vi "evalPerf.vi"(8 "error in (no error)":errorcluster, 11 "removeTempDir":bool=TRUE) -> (0 "error out":errorcluster, 3 "totalTimeInSec":dbl)   [LabVIEW 2018]
doc: "Evaluate the performance. The total used time will show on the panel."
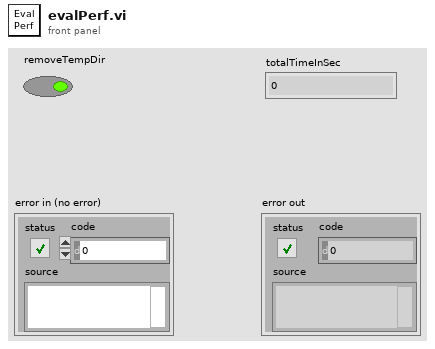
[diagram p1: front panel]
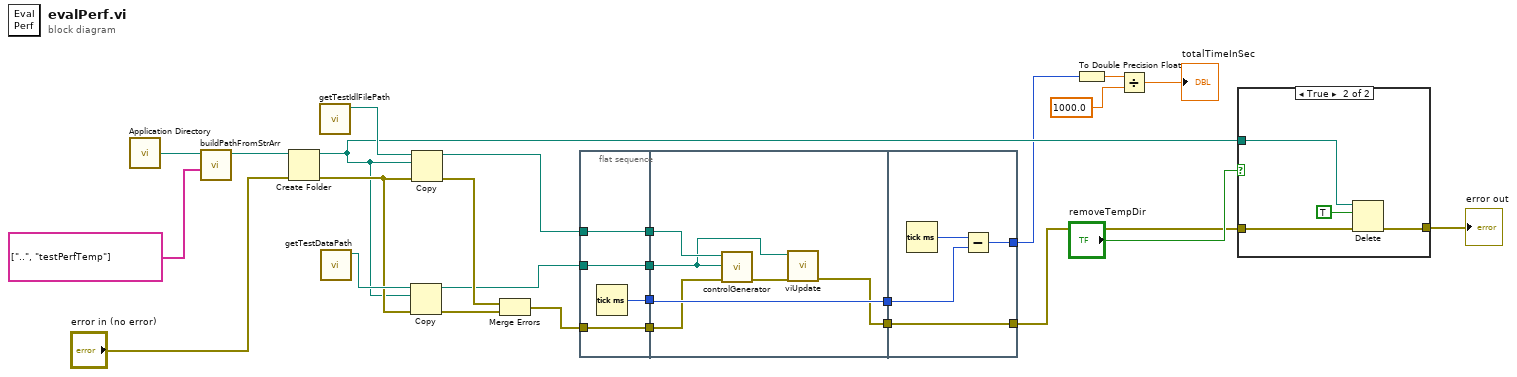
[diagram p0: block diagram]
diagram:
  n1 = call <vilib>:"Application Directory.vi"() -> ("Application Directory"=w26:path)
  n2 = call "buildPathFromStrArr.vi"("String Array"=string[] ["..", "testPerfTemp"], "Root Path"=w26) -> ("Absolute Path"=w24:path)  [unwired: 9 in]
  n3 = Create Folder(path (use dialog)=w24, error in="error in (no error)") -> (created path=w15:path, error out=w20:errorcluster)  [unwired: 1 in, 1 out]
  n4 = call "getTestIdlFilePath.vi"() -> ("testIdlPath"=w22:path)  [unwired: 11 in]
  n5 = call "getTestDataPath.vi"() -> ("testDataPath"=w21:path)  [unwired: 11 in]
  n6 = Copy(8:w20, 10:w15, 11:w21) -> (0:w18:errorcluster, 3:w8:path)  [unwired: 2 in, 1 out]
  n7 = Copy(8:w20, 10:w15, 11:w22) -> (0:w19:errorcluster, 3:w10:path)  [unwired: 2 in, 1 out]
  n8 = Merge Errors(w19, w18) -> (w11:errorcluster)
  n9 = flat-sequence {
    tunnel: [w30] -> w13
    tunnel: [w29] -> w12
    tunnel: w11 -> [w29]
    tunnel: w10 -> [w28]
    tunnel: [w28] -> w9
    tunnel: w8 -> [w27]
    tunnel: [w27] -> w7
    tunnel: [w36] -> w14
    tunnel: w13 -> [w36]
    tunnel: w12 -> [w34]
    tunnel: w9 -> [w33]
    tunnel: w7 -> [w32]
    tunnel: [w31] -> w6
    tunnel: w14 -> [w39]
    tunnel: [w38] -> w5
    tunnel: w6 -> [w38]
    tunnel: [w37] -> w2
    frame #0 {
      n10 = Tick Count (ms)() -> (millisecond timer value=w30:u32)
    }
    frame #1 {
      n11 = call "controlGenerator.vi"("error in (no error)"=w34, "ControlOutputPath"=w32, "ComponentIDLFile"=w33) -> ("error out"=w35:errorcluster)  [unwired: 8 in]
      n12 = call "viUpdate.vi"("error in (no error)"=w35, "OutputPath"=w32) -> ("error out"=w31:errorcluster)  [unwired: 9 in]
    }
    frame #2 {
      n13 = Tick Count (ms)() -> (millisecond timer value=w40:u32)
      n14 = Subtract(x=w40, y=w39) -> (x-y=w37:u32)
    }
  }
  n15 = To Double Precision Float(number=w2) -> (double precision float=w3:dbl)
  n16 = Divide(x=w3, y=1000.0) -> (x/y=→"totalTimeInSec":dbl)
  n17 = case shown="True" "removeTempDir" {
    tunnel: w5 -> [w41 w45]
    tunnel: [w41 w44] -> w16
    tunnel: w15 -> [_ w43]
    frame False {
    }
    frame True {
      n18 = Delete(path (use dialog)=w43, entire hierarchy (F)=TRUE, error in=w45) -> (error out=w44:errorcluster)  [unwired: 2 in, 2 out]
    }
  }
  "error out" <- w16
